vi "Homework 2 Programming Assigment.vi"() -> ()   [LabVIEW 2020]
uses:
  <vilib>/express/express analysis/Spectral/Block/exnSpectralBlock spectral measurements power poly.vi
  <vilib>/express/express analysis/Spectral/Block/exnSpectralBlock spectral measurements power DDT.vi
  <vilib>/express/express analysis/Spectral/XNode/ExpressSpectralMeasurementsBlockNode.xnode
panel:
  in  "Cut-Off Frequency":dbl(slide)=100.0 caption="Lower Cut-Off" scale=1.0..999.0
  in  "?":bool
  out "2":dynamicdata(graph)
  out "?":dynamicdata(graph)
  out "Filtered Signal (High-Pass)":dynamicdata(graph)
  out "Raw Signal":dynamicdata(graph)
  out "Channel 2":dynamicdata(graph)
  out "Channel 1":dynamicdata(graph)
  in  "Frequency":dbl(knob) scale=0.5..1000.0
  in  "Frequency":dbl(knob) scale=0.0..1000.0
  in  "Amplitude":dbl(slide) scale=0.5..10.0
  in  "Amplitude":dbl(slide) scale=0.5..10.0
  # "Channel 1"
  # "Channel 2"
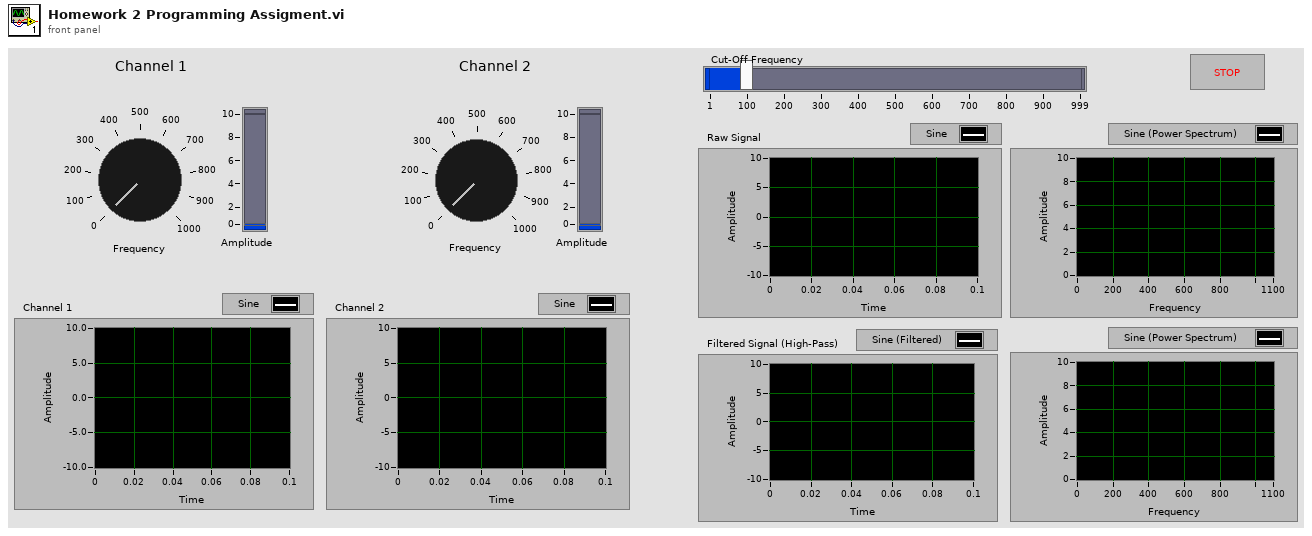
[diagram p1: front panel]
types:
  T1 = cluster{"averaging mode":u16, "weighting mode":u16, "number of averages":u32}
  T2 = cluster{"dB On (F)":bool, "unwrap phase (F)":bool, "convert to degree (F)":bool}
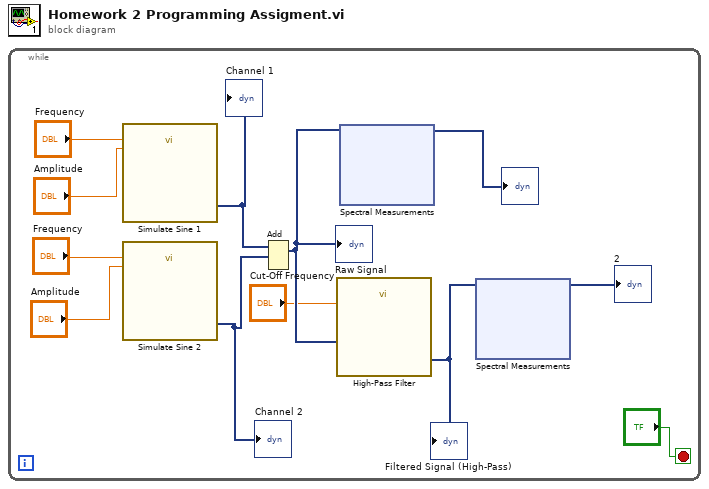
[diagram p0: block diagram]
diagram:
  n1 = while {
    stop <- "?" stop-if-true
    n2 = call "Simulate Sine 1"("Frequency"="Frequency", "Amplitude"="Amplitude") -> ("Sine"=w4:dynamicdata)  [unwired: 12 in, 1 out]
    "Channel 1" <- w4
    n3 = call "Simulate Sine 2"("Frequency"="Frequency", "Amplitude"="Amplitude") -> ("Sine"=w3:dynamicdata)  [unwired: 12 in, 1 out]
    "Channel 2" <- w3
    n4 = Add(1:w3, 2:w4) -> (0:w2:dynamicdata)  [unwired: 1 in, 1 out]
    "Raw Signal" <- w2
    n5 = call "High-Pass Filter"("Lower Cut-Off"="Cut-Off Frequency", "Signal"=w2) -> ("Filtered Signal"=w6:dynamicdata)  [unwired: 8 in, 1 out]
    "Filtered Signal (High-Pass)" <- w6
    n6 = xnode "Spectral Measurements"("Signals"=w2) -> ("Power Spectrum"=→"?":dynamicdata)  [unwired: 1 in, 1 out]
    n7 = xnode "Spectral Measurements"("Signals"=w6) -> ("Power Spectrum"=→"2":dynamicdata)  [unwired: 1 in, 1 out]
  }
